vi "SMD7615 UDP DAQ.vi"(8 "error in (no error)":errorcluster, 9 "StepsPerEncoderInc":i32, 10 "IP":string="192.168.1.30", 11 "connection ID in":refnum<k16>) -> (0 "error out":errorcluster, 1 "DAQ time (ms)":u32, 2 "DAQ Data":T1, 3 "connection ID out":refnum<k16>)   [LabVIEW 2016, in "SMD-7615.lvlib" / "eSCL.lvlib"]
uses:
  eSCL.lvlib
  CTL/Axis Data.ctl
  CTL/Motion IO.ctl
  CTL/Digital Lines (Read).ctl
  CTL/Status.ctl
  CTL/Encoder.ctl
  CTL/Position.ctl
  SMD-7615.lvlib
panel:
  out "CCW Limit":bool
  out "CW Limit":bool
  out "Move Complete":bool
  out "Position":i32
  out "Input Status":string
  out "Velocity":i32
  out "Encoder":i32
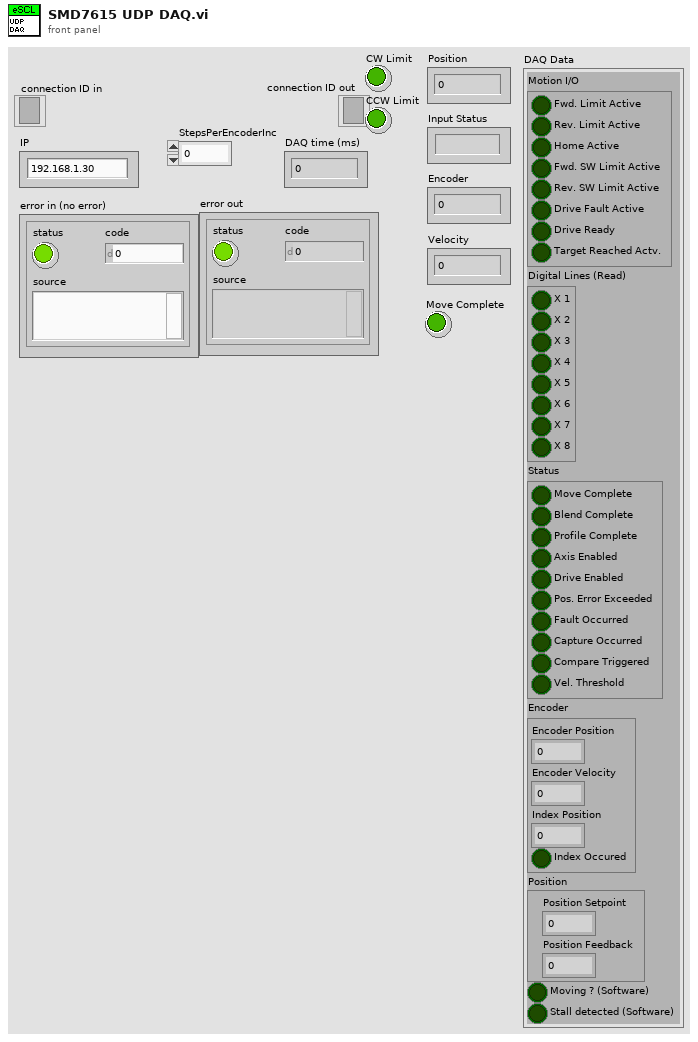
[diagram p1: front panel]
types:
  T1 = typedef "SMD-7615.lvlib/Axis Data.ctl" = cluster{"Motion I/O":T2, "Digital Lines (Read)":T3, "Status":T4, "Encoder":T5, "Position":T6, "Moving ? (Software)":bool, "Stall detected (Software)":bool}
  T2 = typedef "SMD-7615.lvlib/Motion IO.ctl" = cluster{"Fwd. Limit Active":bool, "Rev. Limit Active":bool, "Home Active":bool, "Fwd. SW Limit Active":bool, "Rev. SW Limit Active":bool, "Drive Fault Active":bool, "Drive Ready":bool, "Target Reached Actv.":bool}
  T3 = typedef "SMD-7615.lvlib/Digital Lines (Read).ctl" = cluster{"X 1":bool, "X 2":bool, "X 3":bool, "X 4":bool, "X 5":bool, "X 6":bool, "X 7":bool, "X 8":bool}
  T4 = typedef "SMD-7615.lvlib/Status.ctl" = cluster{"Move Complete":bool, "Blend Complete":bool, "Profile Complete":bool, "Axis Enabled":bool, "Drive Enabled":bool, "Pos. Error Exceeded":bool, "Fault Occurred":bool, "Capture Occurred":bool, "Compare Triggered":bool, "Vel. Threshold":bool}
  T5 = typedef "SMD-7615.lvlib/Encoder.ctl" = cluster{"Encoder Position":dbl, "Encoder Velocity":dbl, "Index Position":dbl, "Index Occured":bool}
  T6 = typedef "SMD-7615.lvlib/Position.ctl" = cluster{"Position Setpoint":dbl, "Position Feedback":dbl}
  T7 = cluster{"[0]":bool, "[1]":bool, "[2]":bool, "[3]":bool, "[4]":bool, "[5]":bool, "[6]":bool, "[7]":bool}
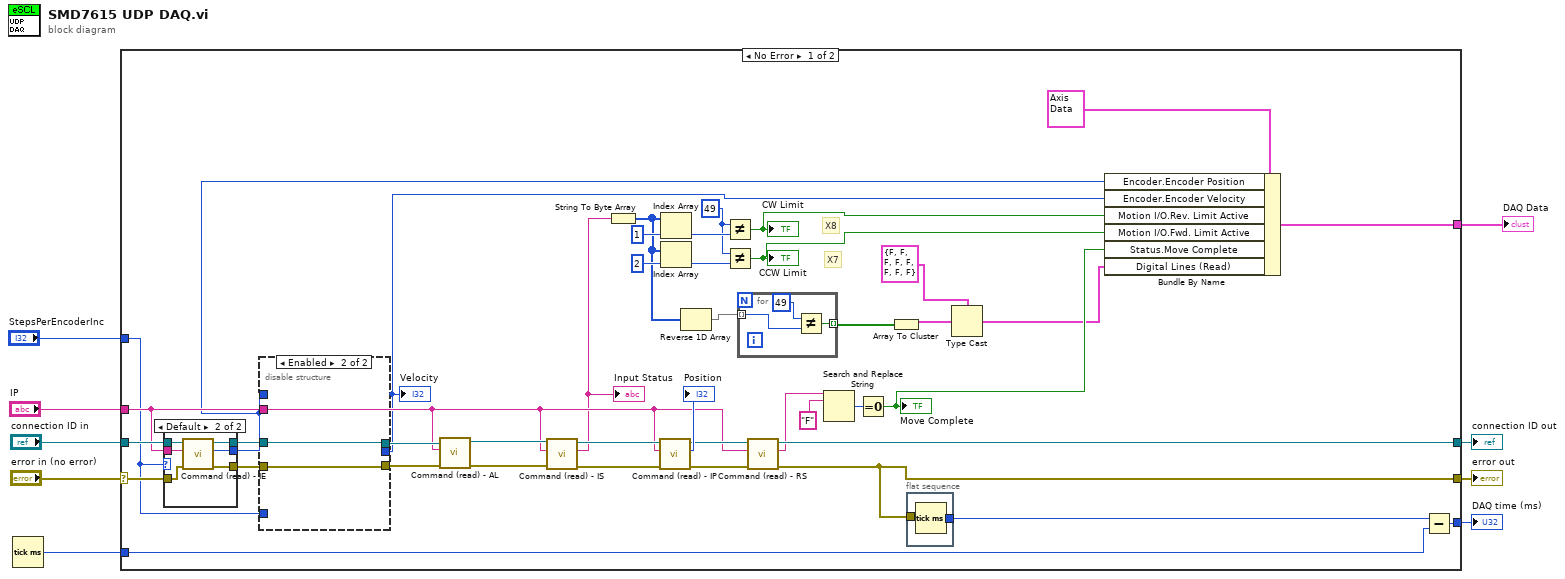
[diagram p0: block diagram]
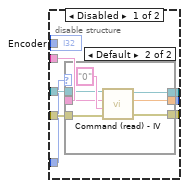
[diagram p2: hidden frame]
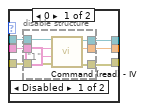
[diagram p3: hidden frame]
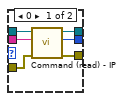
[diagram p5: hidden frame]
diagram:
  n1 = Tick Count (ms)() -> (millisecond timer value=w4:u32)
  n2 = case shown="No Error" "error in (no error)" {
    selector: "error in (no error)" -> [w50 w100]
    tunnel: "connection ID in" -> [w51 w101]
    tunnel: [w40 w101] -> w7
    tunnel: [w27 w100] -> w6
    tunnel: "IP" -> [w37 _]
    tunnel: w4 -> [w25 _]
    tunnel: [w24 _] -> w3
    tunnel: [w13 _] -> w2
    tunnel: "StepsPerEncoderInc" -> [w10 _]
    frame No Error {
      w28 = u8 49 ("x")
      # "X8"
      # "X7"
      n3 = case shown="Default" w10 {
        tunnel: w51 -> [w86 w95]
        tunnel: w50 -> [w89 w94]
        tunnel: [w85 w93] -> w49
        tunnel: [w88 w92] -> w48
        tunnel: w37 -> [w87 w91]
        tunnel: [w84 w90] -> w19
        frame 0 {
          n4 = call "Command (read) - IP.vi"("error in (no error)"=w89, "IP"=w87, "connection ID in"=w86) -> ("error out"=w88:errorcluster, "Position"=w84:i32, "connection ID out"=w85:refnum<k16>)  [unwired: 6 in]
        }
        frame Default {
          n5 = call "Command (read) - IE.vi"("error in (no error)"=w94, "IP"=w91, "connection ID in"=w95) -> ("error out"=w92:errorcluster, "Encoder"=w90:i32, "connection ID out"=w93:refnum<k16>)  [unwired: 6 in]
        }
      }
      n6 = disable-structure shown="Enabled" {
        disable-tunnel: w49 -> [w59 w83]
        disable-tunnel: w48 -> [w58 w82]
        disable-tunnel: [w57 w83] -> w47
        disable-tunnel: [w56 w82] -> w46
        disable-tunnel: w37 -> [w55 _]
        disable-tunnel: w19 -> [w54 _]
        disable-tunnel: [w53 _] -> w18
        disable-tunnel: w10 -> [w52 _]
        frame Disabled {
          n7 = case shown="Default" w52 {
            tunnel: w59 -> [w61 w80]
            tunnel: w58 -> [w62 w79]
            tunnel: [w63 w78] -> w57
            tunnel: [w65 w77] -> w56
            tunnel: w55 -> [w60 w76]
            tunnel: [w64 w75] -> w53
            frame 0 {
              n8 = disable-structure shown="Disabled" {
                disable-tunnel: [w72 w73] -> w65
                disable-tunnel: [w71 _] -> w64
                disable-tunnel: [w70 w74] -> w63
                disable-tunnel: w62 -> [w69 w73]
                disable-tunnel: w61 -> [w68 w74]
                disable-tunnel: w60 -> [w67 _]
                frame Disabled {
                  n9 = call "Command (read) - IV.vi"("error in (no error)"=w69, "Paremeter"="1", "IP"=w67, "connection ID in"=w68) -> ("error out"=w72:errorcluster, "Velocity"=w71:dbl, "connection ID out"=w70:refnum<k16>)  [unwired: 5 in]
                }
                frame Enabled {
                }
              }
            }
            frame Default {
              n10 = call "Command (read) - IV.vi"("error in (no error)"=w79, "Paremeter"="0", "IP"=w76, "connection ID in"=w80) -> ("error out"=w77:errorcluster, "Velocity"=w75:dbl, "connection ID out"=w78:refnum<k16>)  [unwired: 5 in]
            }
          }
          "Encoder" <- w54
        }
        frame Enabled {
        }
      }
      "Velocity" <- w18
      n11 = call "Command (read) - AL.vi"("error in (no error)"=w46, "IP"=w37, "connection ID in"=w47) -> ("error out"=w44:errorcluster, "connection ID out"=w45:refnum<k16>)  [unwired: 6 in, 1 out]
      n12 = call "Command (read) - IS.vi"("error in (no error)"=w44, "IP"=w37, "connection ID in"=w45) -> ("error out"=w42:errorcluster, "Input Status"=w33:string, "connection ID out"=w43:refnum<k16>)  [unwired: 6 in]
      "Input Status" <- w33
      n13 = String To Byte Array(string=w33) -> (unsigned byte array=w11:u8[])
      n14 = call "Command (read) - IP.vi"("error in (no error)"=w42, "IP"=w37, "connection ID in"=w43) -> ("error out"=w38:errorcluster, "Position"=→"Position":i32, "connection ID out"=w39:refnum<k16>)  [unwired: 6 in]
      n15 = Index Array(array=w11, index=1) -> (element=w30:u8)
      n16 = Index Array(array=w11, index=2) -> (element=w29:u8)
      n17 = Reverse 1D Array(array=w11) -> (reversed array=w12:u8[])
      n18 = Not Equal?(x=w28, y=w30) -> (x != y?=w17:bool)
      "CW Limit" <- w17
      n19 = Not Equal?(x=w28, y=w29) -> (x != y?=w16:bool)
      "CCW Limit" <- w16
      n20 = for {
        tunnel: w12 -> [w97] mode=indexing
        tunnel: [w96] -> w23 mode=indexing
        n21 = Not Equal?(x=u8 49, y=w97) -> (x != y?=w96:bool)
      }
      n22 = call "Command (read) - RS.vi"("error in (no error)"=w38, "IP"=w37, "connection ID in"=w39) -> ("error out"=w27:errorcluster, "Status"=w34:string, "connection ID out"=w40:refnum<k16>)  [unwired: 6 in]
      n23 = Search and Replace String(input string=w34, search string="F") -> (number of replacements=w35:i32)  [unwired: 6 in, 3 out]
      n24 = Equal To 0?(x=w35) -> (x = 0?=w15:bool)
      "Move Complete" <- w15
      n25 = Array To Cluster(array=w23) -> (cluster=w22:T7)
      n26 = flat-sequence {
        tunnel: w27 -> [_]
        tunnel: [w99] -> w26
        frame #0 {
          n27 = Tick Count (ms)() -> (millisecond timer value=w99:u32)
        }
      }
      n28 = Type Cast(type=T3 {"X 1"=FALSE, "X 2"=FALSE, "X 3"=FALSE, "X 4"=FALSE, "X 5"=FALSE, "X 6"=FALSE, "X 7"=FALSE, "X 8"=FALSE} ("Digital Lines (Read)"), x=w22) -> (*(type *) &x=w14:T3)
      n29 = Bundle By Name(cluster=T1 {"Motion I/O"={"Fwd. Limit Active"=FALSE, "Rev. Limit Active"=FALSE, "Home Active"=FALSE, "Fwd. SW Limit Active"=FALSE, "Rev. SW Limit Active"=FALSE, "Drive Fault Active"=FALSE, "Drive Ready"=FALSE, "Target Reached Actv."=FALSE}, "Digital Lines (Read)"={"X 1"=FALSE, "X 2"=FALSE, "X 3"=FALSE, "X 4"=FALSE, "X 5"=FALSE, "X 6"=FALSE, "X 7"=FALSE, "X 8"=FALSE}, "Status"={"Move Complete"=FALSE, "Blend Complete"=FALSE, "Profile Complete"=FALSE, "Axis Enabled"=FALSE, "Drive Enabled"=FALSE, "Pos. Error Exceeded"=FALSE, "Fault Occurred"=FALSE, "Capture Occurred"=FALSE, "Compare Triggered"=FALSE, "Vel. Threshold"=FALSE}, "Encoder"={"Encoder Position"=0.0, "Encoder Velocity"=0.0, "Index Position"=0.0, "Index Occured"=FALSE}, "Position"={"Position Setpoint"=0.0, "Position Feedback"=0.0}, "Moving ? (Software)"=FALSE, "Stall detected (Software)"=FALSE} ("Axis Data"), "Encoder.Encoder Position"=w19, "Encoder.Encoder Velocity"=w18, "Motion I/O.Rev. Limit Active"=w17, "Motion I/O.Fwd. Limit Active"=w16, "Status.Move Complete"=w15, "Digital Lines (Read)"=w14) -> (w13:T1)
      n30 = Subtract(x=w26, y=w25) -> (x-y=w24:u32)
    }
    frame Error {
    }
  }
  "connection ID out" <- w7
  "error out" <- w6
  "DAQ time (ms)" <- w3
  "DAQ Data" <- w2
